vi "get_distance.BAK.vi"(11 "NXT":T1={"Hardware"="NXT", "Flattened String"=""}) -> (0 "Distance (cm)":dbl, 3 "NXT 2":T1={"Hardware"="NXT", "Flattened String"=""})   [LabVIEW 2012]
uses:
  <vilib>/NXT/Subs/LVHSConnector.ctl
  <vilib>/NXT/Block Support/NXT_InputPort.ctl
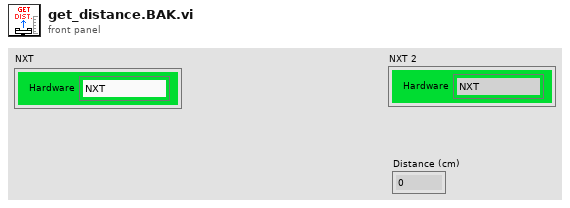
[diagram p1: front panel]
types:
  T1 = typedef "LVHSConnector.ctl" = cluster{"Hardware":string, "Flattened String":string}
  T2 = typedef "NXT_InputPort.ctl" = u8
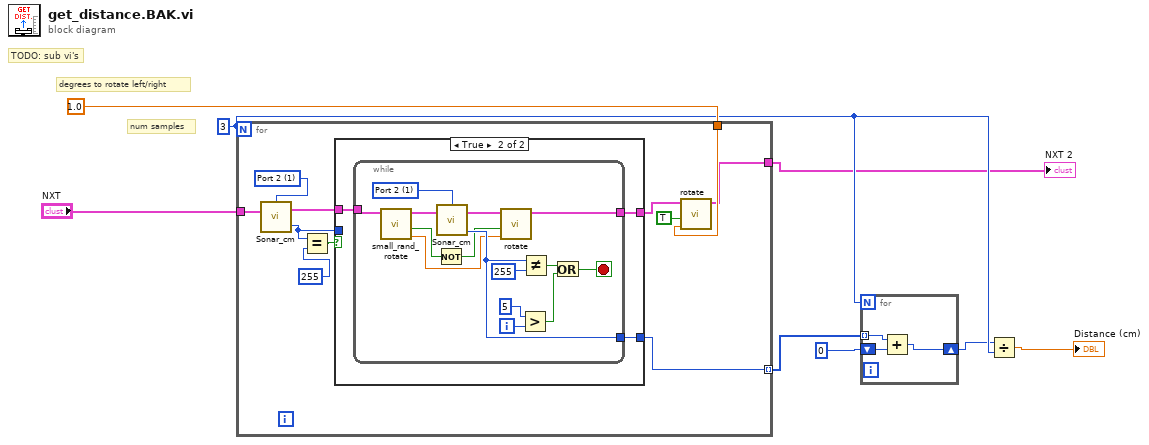
[diagram p0: block diagram]
diagram:
  w4 = 3 ("Angle of Rotation (360)")
  # "num samples"
  # "TODO: sub vi's"
  # "degrees to rotate left/right"
  n1 = for {
    N: w4 -> [_]
    tunnel: [w18] -> w6 mode=indexing
    tunnel: 1.0 ("degrees to  rotate") -> [w15]
    tunnel: [w14] -> w2
    tunnel: "NXT" -> [w13]
    w10 = T2 1 items=["Port 1", "Port 2", "Port 3", "Port 4"] ("Port (Port 4)")
    n2 = call <vilib>:"Sonar_cm.vi"("NXT"=w13, "Port (Port 4)"=w10) -> ("Distance (cm)"=w9:i16, "NXT"=w12:T1)  [unwired: 1 in]
    n3 = Equal?(x=w9, y=255 ("Angle of Rotation (360)")) -> (x = y?=w19:bool)
    n4 = case shown="True" w19 {
      tunnel: [w21 w24] -> w18
      tunnel: [w20 w23] -> w17
      tunnel: w12 -> [w20 w22]
      tunnel: w9 -> [w21 _]
      frame False {
      }
      frame True {
        n5 = while {
          tunnel: [w32] -> w24
          tunnel: [w28] -> w23
          tunnel: w22 -> [w25]
          i -> [w38]
          stop <- w33 stop-if-true
          w37 = T2 1 items=["Port 1", "Port 2", "Port 3", "Port 4"] ("Port (Port 4)")
          n6 = call "small_rand_rotate.vi"("NXT 2"=w25) -> ("degrees rotated"=w30:dbl, "right(T)/left(F)"=w26:bool, "NXT"=w31:T1)  [unwired: 8 in]
          n7 = Not(x=w26) -> (.not. x?=w27:bool)
          n8 = call <vilib>:"Sonar_cm.vi"("NXT"=w31, "Port (Port 4)"=w37) -> ("Distance (cm)"=w32:i16, "NXT"=w29:T1)  [unwired: 1 in]
          n9 = call "rotate.vi"("degrees to  rotate"=w30, "right(T)/left(F)"=w27, "NXT 2"=w29) -> ("NXT"=w28:T1)  [unwired: 8 in]
          n10 = Greater?(x=5, y=w38) -> (0:w35:bool)
          n11 = Not Equal?(x=w32, y=255 ("Angle of Rotation (360)")) -> (x != y?=w34:bool)
          n12 = Or(x=w34, y=w35) -> (x .or. y?=w33:bool)
        }
      }
    }
    n13 = call "rotate.vi"("degrees to  rotate"=w15, "right(T)/left(F)"=TRUE, "NXT 2"=w17) -> ("NXT"=w14:T1)  [unwired: 8 in]
  }
  "NXT 2" <- w2
  n14 = for {
    N: w4 -> [_]
    tunnel: w6 -> [w42] mode=indexing
    shift-right: [w40] -> w3
    shift-left: 0 ("Angle of Rotation (360)") -> [w41]
    n15 = Add(x=w42, y=w41) -> (x+y=w40:i32)
  }
  n16 = Divide(x=w3, y=w4) -> (x/y=→"Distance (cm)":dbl)
